vi "Start.vi"(8 "error in":errorcluster, 11 "Control Load CFG in":refnum<class "EL Control Load CFG.lvclass">) -> (0 "error out":errorcluster, 3 "Control Load CFG out":refnum<class "EL Control Load CFG.lvclass">)   [LabVIEW 2024, in "EL Control Load CFG.lvclass"]
uses:
  EL Control Load CFG.lvclass
  SCPI PE Input.ctl
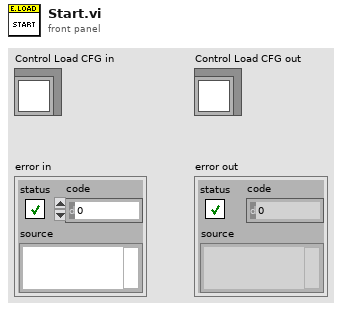
[diagram p1: front panel]
types:
  T1 = typedef "SCPI PE Input.ctl" = cluster{"Action":enum16{"Write", "Query"}, "SCPI":string}
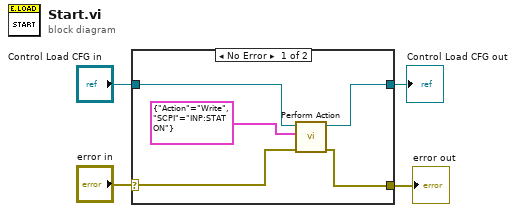
[diagram p0: block diagram]
diagram:
  n1 = case shown="No Error" "error in" {
    selector: "error in" -> [w5 w11]
    tunnel: [w9 w11] -> w4
    tunnel: "Control Load CFG in" -> [w8 w10]
    tunnel: [w7 w10] -> w2
    frame No Error {
      n2 = call-dynamic "Perform Action.vi"("error in"=w5, "Input"=T1 {"Action"=enum."Write", "SCPI"="INP:STAT ON"} ("PE Input"), "Control Load CFG in"=w8) -> ("error out"=w9:errorcluster, "Control Load CFG out"=w7:refnum<class "EL Control Load CFG.lvclass">)  [unwired: 6 in, 1 out]
    }
    frame Error {
    }
  }
  "error out" <- w4
  "Control Load CFG out" <- w2
